vi "read_params.vi"(8 "error in (no error)":errorcluster, 11 "PCA in":refnum<class "PCA.lvclass">) -> (0 "error out":errorcluster, 2 "params":T1={"n_components"={"n_components_type"="None", "n_components_int"=0, "n_components_float"=0.0}, "copy"=TRUE, "whiten"=FALSE, "svd_solver"="auto", "tol"=0.0, "iterated_power"={"iterated_power_type"="auto", "iterated_power_int"=0.0}, "random_state"=0.0}, 3 "PCA out":refnum<class "PCA.lvclass">)   [LabVIEW 2020, in "PCA.lvclass"]
uses:
  PCA.lvclass
  Controls/pca_params.ctl
  PCA.lvclass/PCA.ctl
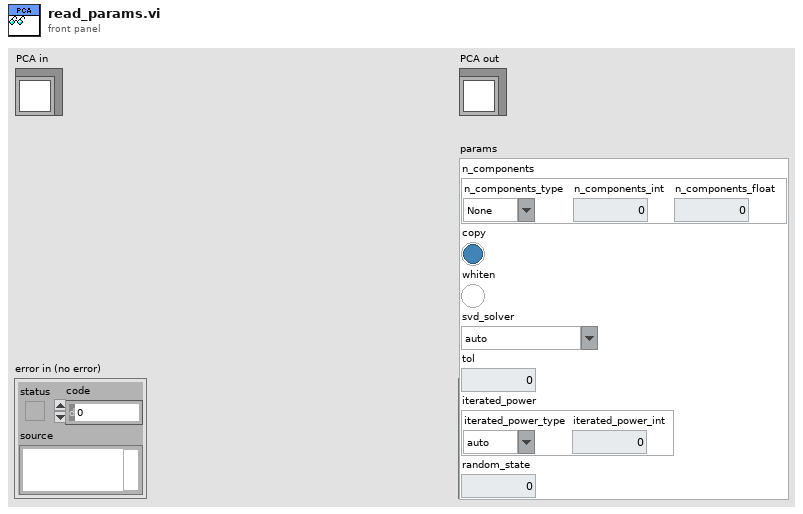
[diagram p1: front panel]
types:
  T1 = typedef "pca_params.ctl" = cluster{"n_components":cluster{"n_components_type":string, "n_components_int":i32, "n_components_float":dbl}, "copy":bool, "whiten":bool, "svd_solver":string, "tol":dbl, "iterated_power":cluster{"iterated_power_type":string, "iterated_power_int":dbl}, "random_state":dbl}
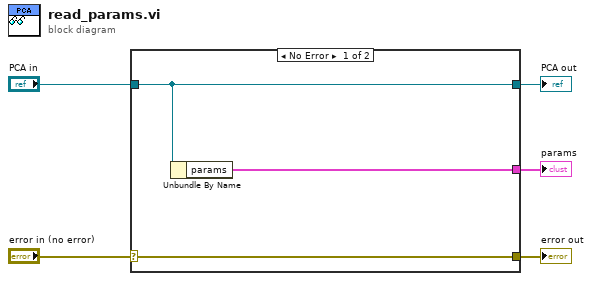
[diagram p0: block diagram]
diagram:
  n1 = case shown="No Error" "error in (no error)" {
    selector: "error in (no error)" -> [w8 w9]
    tunnel: [w8 w9] -> w4
    tunnel: [w7 w10] -> w2
    tunnel: "PCA in" -> [w7 w10]
    tunnel: [w6 _] -> w1
    frame No Error {
      n2 = Unbundle By Name(w7) -> ("params"=w6:T1)
    }
    frame Error {
    }
  }
  "error out" <- w4
  "PCA out" <- w2
  "params" <- w1
